vi "Leybold TURBOVAC Configure And Operate.vi"() -> ()   [LabVIEW 2019]
doc: "Example VI to demonstrate the use of the Oerlikon Leybold TMP driver."
uses:
  <instrlib>/Leybold TURBOVAC/Public/Ctl/Converter Type Control.ctl
  <instrlib>/Leybold TURBOVAC/Leybold TURBOVAC.lvlib
panel:
  in  "Nominal frequency (1000)":u16=1000 max=700
  in  "Change nominal frequency (F: off)":bool
  in  "Converter Type\n(180: Turbovac 350/450 i)":T1=187 items=["Turbovac 350/450 i"=180, "Turbovac 350/450 i with optional interface"=181, "Turbovac 350/450 iX"=182, "Turbovac  90/250 i"=190, "Turbovac  90/250 with optional interface"=191, "Turbovac  90/250 iX"=192, "Turbovac  850/950 i"=195, "Turbovac  850/950 i with optional interface"=196, "Turbovac  850/950 iX"=197, "Turbovac 1350/1450 i"=185, "Turbovac 1350/1450 i with optional interface"=186, "Turbovac 1350/1450 iX"=187]
  in  "Enable Standby (F: off)":bool
  in  "Enable Remote Control (F: off)":bool
  in  "Operate pump (F: off)":bool
  out "Warnings / Errors":string
  out "Status values":T2
  out "Status word":T3
  in  "stop":bool
  in  "Converter address (0)":u8
  in  "VISA resource name":refnum<visa-resource-name>="COM44"
  # "© 2020 Leybold.  ALL RIGHTS RESERVED."
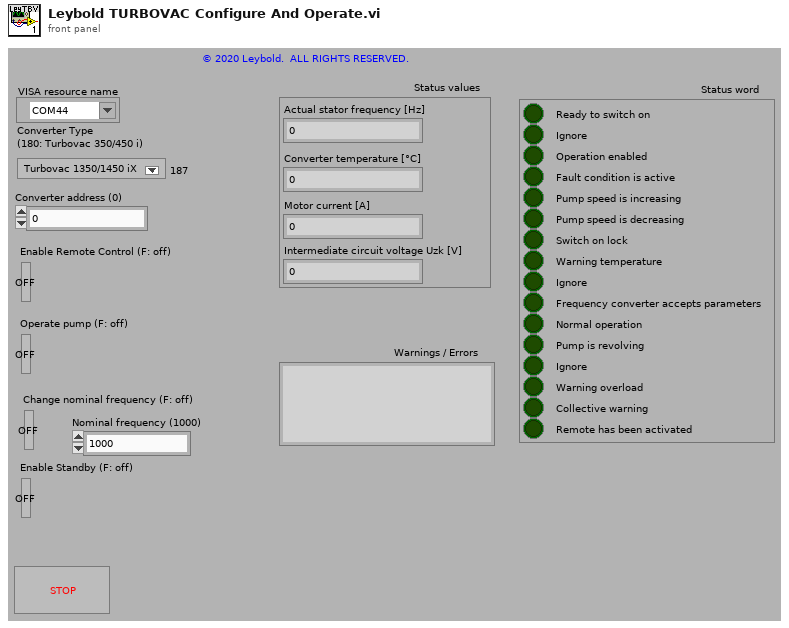
[diagram p1: front panel]
types:
  T1 = typedef "Leybold TURBOVAC.lvlib/Converter Type Control.ctl" = u16
  T2 = cluster{"Actual stator frequency [Hz]":u16, "Converter temperature [°C]":u16, "Motor current [A]":dbl, "Intermediate circuit voltage Uzk [V]":dbl}
  T3 = cluster{"Ready to switch on":bool, "Ignore":bool, "Operation enabled":bool, "Fault condition is active":bool, "Pump speed is increasing":bool, "Pump speed is decreasing":bool, "Switch on lock":bool, "Warning temperature":bool, "Ignore":bool, "Frequency converter accepts parameters":bool, "Normal operation":bool, "Pump is revolving":bool, "Ignore":bool, "Warning overload":bool, "Collective warning":bool, "Remote has been activated":bool}
  T4 = typedef "Leybold TURBOVAC.lvlib/Device Parameters Indicator.ctl" = cluster{"Length of data block":u8, "Converter address":u8, "Converter type":T5, "PZD1":u16, "PZD2":u16}
  T5 = typedef "Leybold TURBOVAC.lvlib/Converter Type Indicator.ctl" = u16
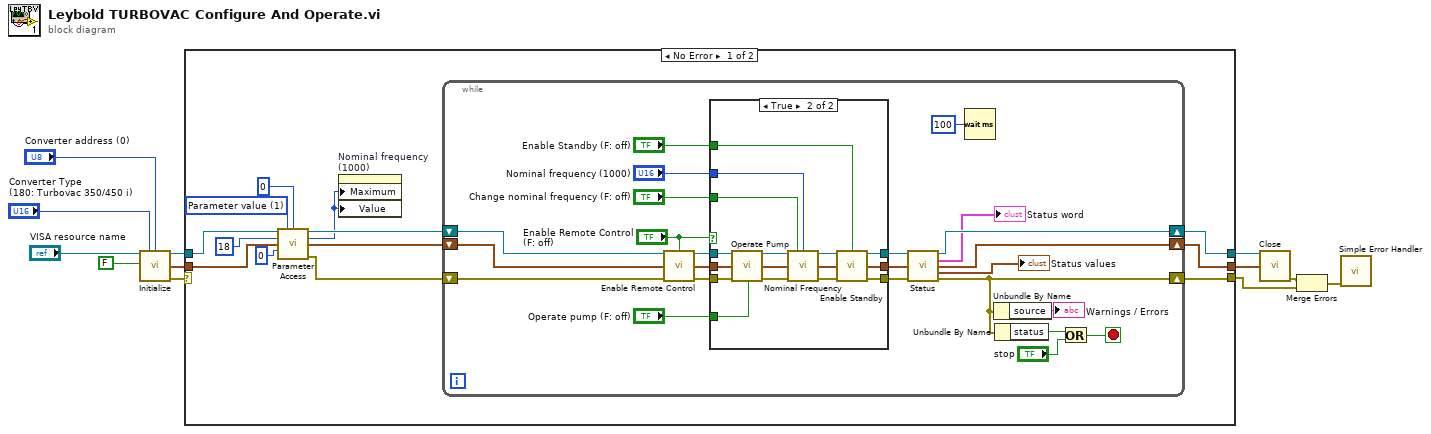
[diagram p0: block diagram]
diagram:
  n1 = call <instrlib>:"Initialize.vi"("VISA resource name"="VISA resource name", "Converter Type\n(180: Turbovac 350/450 i)"="Converter Type\n(180: Turbovac 350/450 i)", "Converter address (0)"="Converter address (0)", "ID Query? (T: Yes)"=FALSE) -> ("VISA resource name out"=w8:refnum<visa-resource-name>, "Device parameters out"=w7:T4, "error out"=w6:errorcluster)  [unwired: 9 in]
  n2 = case shown="No Error" w6 {
    selector: w6 -> [_ w69]
    tunnel: w8 -> [w25 w70]
    tunnel: w7 -> [w24 w71]
    tunnel: [w18 w70] -> w5
    tunnel: [w17 w71] -> w4
    tunnel: [w15 w69] -> w2
    frame No Error {
      w21 = u8 1 items=["Do nothing"=0, "Parameter value"=1, "Write 16 bit value"=2, "Write 32 bit value"=3, "Field value requested"=6, "Write 16 bit field value"=7, "Write 32 bit field value"=8, "Request No. of field elements"=9] ("Type of parameter access (1: Parameter value)")
      n3 = call <instrlib>:"Parameter Access.vi"("VISA resource name"=w25, "Type of parameter access (1: Parameter value)"=w21, "PWE (0)"=0, "PKE-PM No. (1)"=u16 18, "Device parameters"=w24, "Index (0)"=u16 0) -> ("VISA resource name out"=w20:refnum<visa-resource-name>, "PWE out"=w14:i32, "Device parameters out"=w19:T4, "error out"=w16:errorcluster)  [unwired: 6 in]
      n4 = property on="Nominal frequency (1000)" class="DigNum (strict)"("Maximum"=w14, "Value"=w14) -> ()  [unwired: 2 in, 2 out]
      n5 = while {
        shift-right: [w34] -> w17
        shift-left: w19 -> [w37]
        shift-right: [w26] -> w15
        shift-left: w16 -> [w41]
        shift-right: [w46] -> w18
        shift-left: w20 -> [w38]
        stop <- w49 stop-if-true
        n6 = call <instrlib>:"Enable Remote Control.vi"("VISA resource name"=w38, "Enable Remote Control (F: off)"="Enable Remote Control (F: off)", "Device parameters"=w37, "error in (no error)"=w41) -> ("VISA resource name out"=w39:refnum<visa-resource-name>, "Device parameters out"=w36:T4, "error out"=w40:errorcluster)  [unwired: 9 in]
        n7 = case shown="True" "Enable Remote Control (F: off)" {
          tunnel: w40 -> [w50 w68]
          tunnel: w39 -> [w52 w67]
          tunnel: w36 -> [w51 w66]
          tunnel: "Operate pump (F: off)" -> [_ w65]
          tunnel: [w50 w64] -> w33
          tunnel: [w51 w63] -> w32
          tunnel: [w52 w62] -> w31
          tunnel: "Enable Standby (F: off)" -> [_ w61]
          tunnel: "Change nominal frequency (F: off)" -> [_ w54]
          tunnel: "Nominal frequency (1000)" -> [_ w53]
          frame False {
          }
          frame True {
            n8 = call <instrlib>:"Operate Pump.vi"("VISA resource name"=w67, "Operate pump (F: off)"=w65, "Device parameters"=w66, "error in (no error)"=w68) -> ("VISA resource name out"=w60:refnum<visa-resource-name>, "Device parameters out"=w58:T4, "error out"=w59:errorcluster)  [unwired: 9 in]
            n9 = call <instrlib>:"Nominal Frequency.vi"("VISA resource name"=w60, "Change nominal frequency (F: off)"=w54, "Nominal frequency (1000)"=w53, "Device parameters"=w58, "error in (no error)"=w59) -> ("VISA resource name out"=w56:refnum<visa-resource-name>, "Device parameters out"=w55:T4, "error out"=w57:errorcluster)  [unwired: 8 in]
            n10 = call <instrlib>:"Enable Standby.vi"("VISA resource name"=w56, "Activate Standy (F: off)"=w61, "Device parameters"=w55, "error in (no error)"=w57) -> ("VISA resource name out"=w62:refnum<visa-resource-name>, "Device parameters out"=w63:T4, "error out"=w64:errorcluster)  [unwired: 9 in]
          }
        }
        n11 = call <instrlib>:"Status.vi"("VISA resource name"=w31, "Device parameters"=w32, "error in (no error)"=w33) -> ("VISA resource name out"=w46:refnum<visa-resource-name>, "Status word"=→"Status word":T3, "Device parameters out"=w34:T4, "Status values"=→"Status values":T2, "error out"=w26:errorcluster)  [unwired: 8 in]
        n12 = Wait (ms)(milliseconds to wait=u32 100) -> ()  [unwired: 1 out]
        n13 = Unbundle By Name(w26) -> ("source"=→"Warnings / Errors":string)
        n14 = Unbundle By Name(w26) -> ("status"=w47:bool)
        n15 = Or(x=w47, y="stop") -> (x .or. y?=w49:bool)
      }
    }
    frame Error {
    }
  }
  n16 = call <instrlib>:"Close.vi"("VISA resource name"=w5, "Device Parameters"=w4) -> ("error out"=w11:errorcluster)  [unwired: 13 in]
  n17 = Merge Errors(w11, w2) -> (w3:errorcluster)
  n18 = call <vilib>:"Simple Error Handler.vi"("error in (no error)"=w3) -> ()  [unwired: 4 in, 5 out]
